vi "挥发酚测量数据储存.vi"   [LabVIEW 2016, in "挥发酚.lvlib"]
uses:
  <vilib>/ptbypt/NI_PtbyPt.lvlib
types:
  T1 = cluster{"时间标识":timestamp, "监测值":sgl, "单位":u16, "数据标识":string, "因子编码":u32, "标样参考值":sgl, "X0":sgl, "X^2":sgl, "X":sgl, "B 2":sgl, "跨度值":sgl, "量程":sgl}
  T2 = enum16{"维护数据", "水样测试", "标样核查", "零点核查", "跨度核查", "空白测试", "平行样测试", "加标回收", "空白校准", "标样校准", "初始化（清洗）"}
  T3 = cluster{"系统时间":timestamp, "工作状态":u16, "测量模式":enum16{"待机", "连续模式", "周期模式", "定点模式", "受控模式", "手动模式"}, "告警代码":u16, "故障代码":u16, "日志代码":u16, "软件版本":u16, "测量间隔":u16, "消解实时温度":dbl, "校准间隔（天）":u16, "校准间隔（时）":u16, "周期测量时间（23_16）":u16, "周期测量时间（15_0）":u16, "清洗周期（次数）":u16, "运行模式":u16, "自动校准状态":u16, "自动清洗状态":u16}
  T4 = enum16{"水样测试", "标样核查", "跨度核查", "零点核查", "空白测试", "平行样测试", "加标回收", "空白校准", "标样1校准", "标样2校准"}[]
  T5 = cluster{"运行模式":enum16{"维护模式", "常规模式", "应急模式", "质控模式", "性能测试"}, "质控频次":enum16{"关闭", "每天", "星期一", "星期二", "星期三", "星期四", "星期五", "星期六", "星期日"}, "空白核查时间":u16, "跨度核查时间":u16, "测量间隔":u16}
  T6 = cluster{"因子编码":u32, "单位":u16, "标样2参考值":sgl, "水样数据时间":timestamp, "水样实测值":sgl, "水样数据标识":string, "标样2数据时间":timestamp, "标样2实测值":sgl, "标样2数据标识":string, "空白数据时间":timestamp, "空白实测值":sgl, "空白数据标识":string, "零点核查数据时间":timestamp, "零点核查实测值":sgl, "零点核查数据标识":string, "跨度核查数据时间":timestamp, "跨度核查实测值":sgl, "跨度核查数据标识":string, "加标回收数据时间":timestamp, "加标回收实测值":sgl, "加标回收数据标识":string, "平行样数据时间":timestamp, "平行样实测值":sgl, "平行样数据标识":string, "标样1参考值":sgl, "标样1数据时间":timestamp, "标样1实测值":sgl, "标样1数据标识":string, "标样核查数据时间":timestamp, "标样核查实测值":sgl, "标样核查数据标识":string}
  T7 = cluster{"跨度值":dbl, "零点标准液浓度":dbl, "跨度标准液浓度":dbl, "标准液标准浓度":dbl, "零点标准液偏差":dbl, "跨度标准液偏差":dbl, "标准液标准偏差":dbl}
  T8 = cluster{"水样数据时间":timestamp, "空白数据时间":timestamp, "零点核查数据时间":timestamp, "跨度核查数据时间":timestamp, "加标回收数据时间":timestamp, "平行样数据时间":timestamp, "标样核查数据时间":timestamp, "标样1数据时间":timestamp, "标样2数据时间":timestamp}
  T9 = cluster{"公式":cluster{"X^2":dbl, "X":dbl, "B":dbl}, "校准":cluster{"校准？":bool, "校准点1-5":u16, "校准浓度":dbl}}
  T10 = cluster{"测量精度":u16, "消解温度":u16, "消解时长":u16, "量程下限":sgl, "量程上限":sgl, "曲线斜率K":sgl, "曲线斜率B":sgl, "标定日期":timestamp, "标液1浓度":sgl, "标液1测量过程值":sgl, "标液2浓度":sgl, "标液2测量过程值":sgl, "标液3浓度":sgl, "标液3测量过程值":sgl, "标液4浓度":sgl, "标液4测量过程值":sgl, "标液5浓度":sgl, "标液5测量过程值":sgl, "线性相关系数":sgl, "试剂余量":u32, "测量滴定值或吸光度":sgl, "标样2校准时间":timestamp, "检出限值":sgl, "校准系数":sgl, "设备系列号":string, "显色温度":u16, "显色时间":u16, "试剂余量1":u16, "试剂余量2":u16, "试剂余量3":u16, "试剂余量4":u16, "试剂余量5":u16, "试剂余量6":u16, "试剂余量7":u16, "试剂余量8":u16, "试剂余量9":u16, "试剂余量10":u16, "当前量程低位":sgl, "当前量程高位":sgl}
  T11 = cluster{"测量量程":sgl, "测量检出限":sgl, "测量精度":sgl, "测量间隔":sgl, "消解温度":sgl, "消解时长":sgl, "三项式系数":sgl, "二次多项式系数":sgl, "曲线斜率":sgl, "曲线截距":sgl, "线性相关系数":sgl, "空白校准时间":timestamp, "标样校准时间":timestamp, "测量信号值":sgl, "稀释倍数":sgl, "量程系数":sgl}
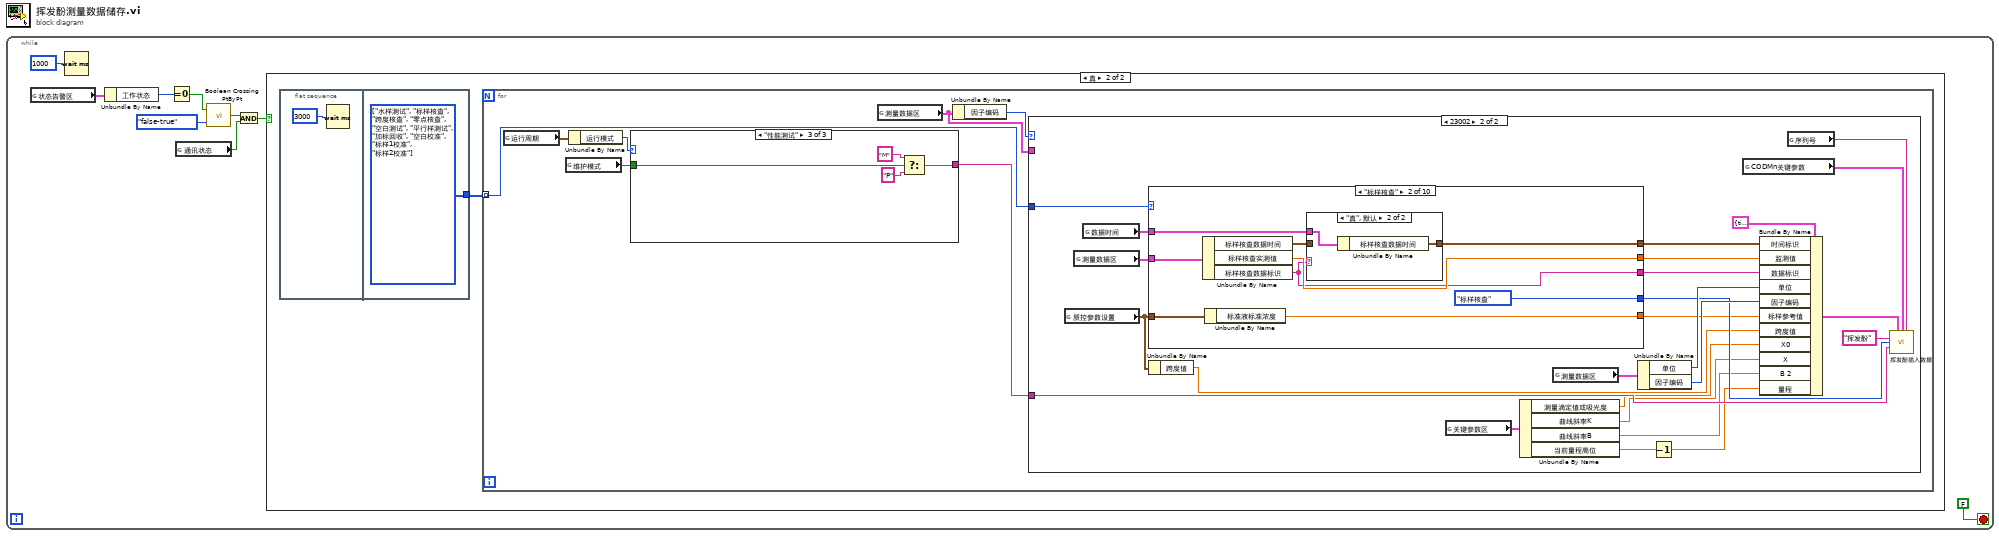
[diagram p0: block diagram]
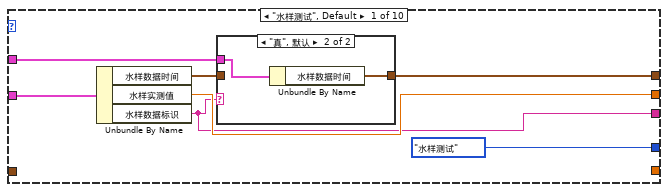
[diagram p4: hidden frame]
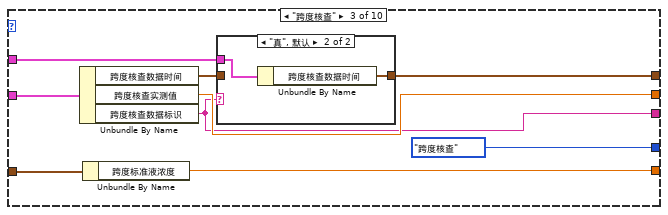
[diagram p7: hidden frame]
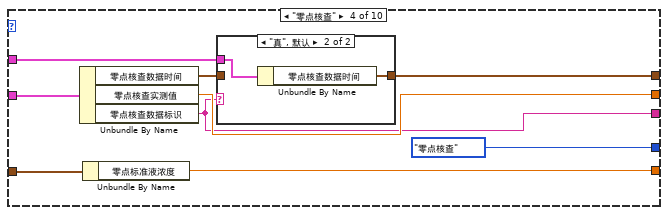
[diagram p9: hidden frame]
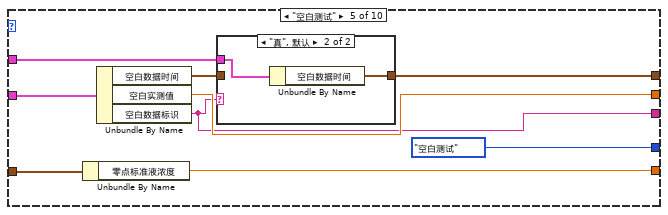
[diagram p11: hidden frame]
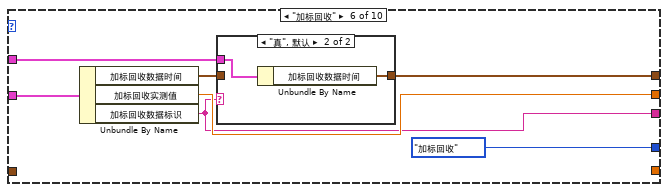
[diagram p13: hidden frame]
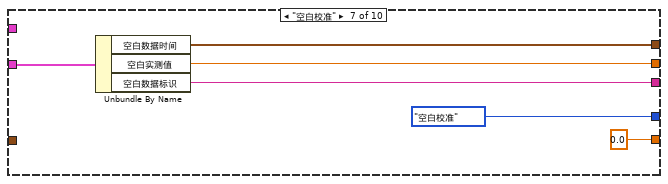
[diagram p15: hidden frame]
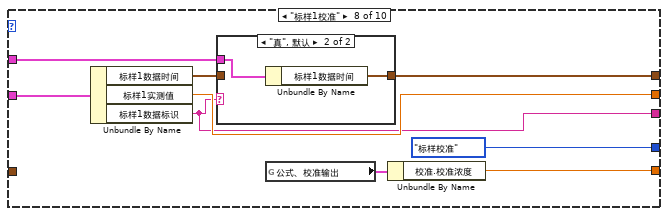
[diagram p16: hidden frame]
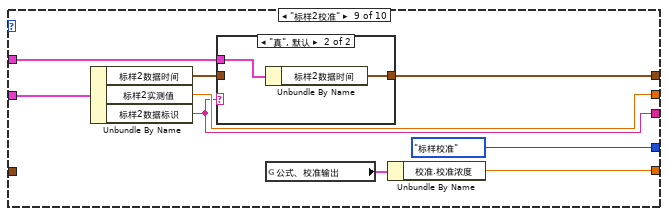
[diagram p18: hidden frame]
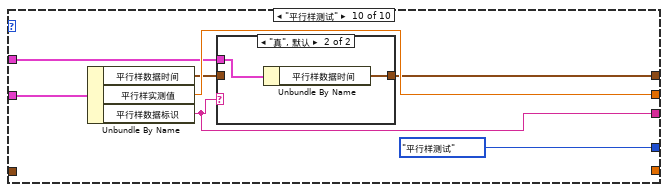
[diagram p20: hidden frame]
diagram:
  n1 = while {
    stop <- FALSE stop-if-true
    n2 = global read "VAR挥发酚全局变量.vi" "状态告警区"() -> (w5:T3)
    n3 = Wait (ms)(milliseconds to wait=u32 1000 ("等待时间（毫秒）")) -> ()  [unwired: 1 out]
    n4 = Unbundle By Name(w5) -> ("工作状态"=w4:u16)
    n5 = Equal To 0?(x=w4) -> (x = 0?=w6:bool)
    n6 = global read "VAR挥发酚全局变量.vi" "通讯状态"() -> (w2:bool)
    n7 = call <vilib>:"Boolean Crossing PtByPt.vi"("direction"=enum16{"either", "false-true", "true-false"}."false-true", "input"=w6) -> ("crossing"=w3:bool)  [unwired: 1 in]
    n8 = And(x=w3, y=w2) -> (x .and. y?=w1:bool)
    n9 = case shown="真" w1 {
      frame False {
      }
      frame True {
        n10 = flat-sequence {
          tunnel: [w12] -> w10
          frame #0 {
            n11 = Wait (ms)(milliseconds to wait=u32 3000 ("等待时间（毫秒）")) -> ()  [unwired: 1 out]
          }
          frame #1 {
            w12 = T4 [enum."水样测试", enum."标样核查", enum."跨度核查", enum."零点核查", enum."空白测试", enum."平行样测试", enum."加标回收", enum."空白校准", enum."标样1校准", enum."标样2校准"] items=["水样测试", "标样核查", "跨度核查", "零点核查", "空白测试", "平行样测试", "加标回收", "空白校准", "标样1校准", "标样2校准"]
          }
        }
        n12 = for {
          tunnel: w10 -> [w18] mode=indexing
          n13 = global read "挥发酚断电保存全局变量.vi" "运行周期"() -> (w17:T5)
          n14 = global read "挥发酚断电保存全局变量.vi" "维护模式"() -> (w13:bool)
          n15 = Unbundle By Name(w17) -> ("运行模式"=w14:enum16{"维护模式", "常规模式", "应急模式", "质控模式", "性能测试"})
          n16 = case shown="\"性能测试\"" w14 {
            tunnel: ["M" ("数据标记表") w154 w162] -> w19
            tunnel: w13 -> [_ w157 w164]
            frame "维护模式" {
            }
            frame "常规模式", Default {
              n17 = global read "VAR挥发酚全局变量.vi" "手动启动"() -> (w158:bool)
              n18 = case shown="假" w158 {
                tunnel: ["N" ("数据标记表") "hd" ("数据标记表")] -> w156
                frame False {
                }
                frame True {
                }
              }
              n19 = Select(t="M", s=w157, f=w156) -> (s? t:f=w154:string)
            }
            frame "性能测试" {
              n20 = Select(t="M", s=w164, f="P") -> (s? t:f=w162:string)
            }
          }
          n21 = global read "VAR挥发酚全局变量.vi" "测量数据区"() -> (w16:T6)
          n22 = Unbundle By Name(w16) -> ("因子编码"=w15:u32)
          n23 = case shown="23002" w15 {
            tunnel: w16 -> [_ _]
            tunnel: w19 -> [_ w34]
            tunnel: w18 -> [_ w33]
            frame Default {
            }
            frame 23002 {
              n24 = global read "挥发酚断电保存全局变量.vi" "质控参数设置"() -> (w30:T7)
              n25 = global read "VAR挥发酚全局变量.vi" "测量数据区"() -> (w44:T6)
              n26 = global read "挥发酚断电保存全局变量.vi" "数据时间"() -> (w22:T8)
              n27 = case shown="\"标样核查\"" w33 {
                tunnel: w44 -> [w51 w63 w75 w87 w99 w109 w118 w127 w139 w148]
                tunnel: [w45 w55 w69 w81 w91 w103 w117 w121 w131 w143] -> w37
                tunnel: [w49 w62 w74 w86 w98 w107 w116 w126 w138 w147] -> w38
                tunnel: [w47 w57 w67 w79 w93 w106 w115 w119 w134 w145] -> w39
                tunnel: [T2."水样测试" ("测量模式") T2."标样核查" ("测量模式") T2."跨度核查" ("测量模式") T2."零点核查" ("测量模式") T2."空白测试" ("测量模式") T2."加标回收" ("测量模式") T2."空白校准" ("测量模式") T2."标样校准" ("测量模式") T2."标样校准" ("测量模式") T2."平行样测试" ("测量模式")] -> w36
                tunnel: w30 -> [_ w59 w72 w84 w95 _ _ _ _ _]
                tunnel: [_ w60 w71 w83 w96 _ 0.0 ("零点标准液浓度") w124 w136 _] -> w32
                tunnel: w22 -> [w48 w58 w68 w80 w94 w105 _ w122 w132 w146]
                frame "水样测试", Default {
                  n28 = Unbundle By Name(w51) -> ("水样数据时间"=w46:timestamp, "水样实测值"=w49:sgl, "水样数据标识"=w47:string)
                  n29 = case shown="\"真\", 默认" w47 {
                    tunnel: w48 -> [_ w54]
                    tunnel: w46 -> [w52 _]
                    tunnel: [w52 w53] -> w45
                    frame "N" {
                    }
                    frame "真", Default {
                      n30 = Unbundle By Name(w54) -> ("水样数据时间"=w53:timestamp)
                    }
                  }
                }
                frame "标样核查" {
                  n31 = Unbundle By Name(w63) -> ("标样核查数据时间"=w56:timestamp, "标样核查实测值"=w62:sgl, "标样核查数据标识"=w57:string)
                  n32 = Unbundle By Name(w59) -> ("标准液标准浓度"=w60:dbl)
                  n33 = case shown="\"真\", 默认" w57 {
                    tunnel: w58 -> [_ w66]
                    tunnel: w56 -> [w64 _]
                    tunnel: [w64 w65] -> w55
                    frame "N" {
                    }
                    frame "真", Default {
                      n34 = Unbundle By Name(w66) -> ("标样核查数据时间"=w65:timestamp)
                    }
                  }
                }
                frame "跨度核查" {
                  n35 = Unbundle By Name(w75) -> ("跨度核查数据时间"=w70:timestamp, "跨度核查实测值"=w74:sgl, "跨度核查数据标识"=w67:string)
                  n36 = Unbundle By Name(w72) -> ("跨度标准液浓度"=w71:dbl)
                  n37 = case shown="\"真\", 默认" w67 {
                    tunnel: w68 -> [_ w78]
                    tunnel: w70 -> [w76 _]
                    tunnel: [w76 w77] -> w69
                    frame "N" {
                    }
                    frame "真", Default {
                      n38 = Unbundle By Name(w78) -> ("跨度核查数据时间"=w77:timestamp)
                    }
                  }
                }
                frame "零点核查" {
                  n39 = Unbundle By Name(w87) -> ("零点核查数据时间"=w82:timestamp, "零点核查实测值"=w86:sgl, "零点核查数据标识"=w79:string)
                  n40 = Unbundle By Name(w84) -> ("零点标准液浓度"=w83:dbl)
                  n41 = case shown="\"真\", 默认" w79 {
                    tunnel: w80 -> [_ w90]
                    tunnel: w82 -> [w88 _]
                    tunnel: [w88 w89] -> w81
                    frame "N" {
                    }
                    frame "真", Default {
                      n42 = Unbundle By Name(w90) -> ("零点核查数据时间"=w89:timestamp)
                    }
                  }
                }
                frame "空白测试" {
                  n43 = Unbundle By Name(w95) -> ("零点标准液浓度"=w96:dbl)
                  n44 = Unbundle By Name(w99) -> ("空白数据时间"=w92:timestamp, "空白实测值"=w98:sgl, "空白数据标识"=w93:string)
                  n45 = case shown="\"真\", 默认" w93 {
                    tunnel: w94 -> [_ w102]
                    tunnel: w92 -> [w100 _]
                    tunnel: [w100 w101] -> w91
                    frame "N" {
                    }
                    frame "真", Default {
                      n46 = Unbundle By Name(w102) -> ("空白数据时间"=w101:timestamp)
                    }
                  }
                }
                frame "加标回收" {
                  n47 = Unbundle By Name(w109) -> ("加标回收数据时间"=w104:timestamp, "加标回收实测值"=w107:sgl, "加标回收数据标识"=w106:string)
                  n48 = case shown="\"真\", 默认" w106 {
                    tunnel: w105 -> [_ w112]
                    tunnel: w104 -> [w110 _]
                    tunnel: [w110 w111] -> w103
                    frame "N" {
                    }
                    frame "真", Default {
                      n49 = Unbundle By Name(w112) -> ("加标回收数据时间"=w111:timestamp)
                    }
                  }
                }
                frame "空白校准" {
                  n50 = Unbundle By Name(w118) -> ("空白数据时间"=w117:timestamp, "空白实测值"=w116:sgl, "空白数据标识"=w115:string)
                }
                frame "标样1校准" {
                  n51 = Unbundle By Name(w127) -> ("标样1数据时间"=w120:timestamp, "标样1实测值"=w126:sgl, "标样1数据标识"=w119:string)
                  n52 = case shown="\"真\", 默认" w119 {
                    tunnel: w122 -> [_ w130]
                    tunnel: w120 -> [w128 _]
                    tunnel: [w128 w129] -> w121
                    frame "N" {
                    }
                    frame "真", Default {
                      n53 = Unbundle By Name(w130) -> ("标样1数据时间"=w129:timestamp)
                    }
                  }
                  n54 = global read "挥发酚断电保存全局变量.vi" "公式、校准输出"() -> (w123:T9)
                  n55 = Unbundle By Name(w123) -> ("校准.校准浓度"=w124:dbl)
                }
                frame "标样2校准" {
                  n56 = Unbundle By Name(w139) -> ("标样2数据时间"=w133:timestamp, "标样2实测值"=w138:sgl, "标样2数据标识"=w134:string)
                  n57 = case shown="\"真\", 默认" w134 {
                    tunnel: w132 -> [_ w142]
                    tunnel: w133 -> [w140 _]
                    tunnel: [w140 w141] -> w131
                    frame "N" {
                    }
                    frame "真", Default {
                      n58 = Unbundle By Name(w142) -> ("标样2数据时间"=w141:timestamp)
                    }
                  }
                  n59 = global read "挥发酚断电保存全局变量.vi" "公式、校准输出"() -> (w135:T9)
                  n60 = Unbundle By Name(w135) -> ("校准.校准浓度"=w136:dbl)
                }
                frame "平行样测试" {
                  n61 = Unbundle By Name(w148) -> ("平行样数据时间"=w144:timestamp, "平行样实测值"=w147:sgl, "平行样数据标识"=w145:string)
                  n62 = case shown="\"真\", 默认" w145 {
                    tunnel: w146 -> [_ w152]
                    tunnel: w144 -> [w150 _]
                    tunnel: [w150 w151] -> w143
                    frame "N" {
                    }
                    frame "真", Default {
                      n63 = Unbundle By Name(w152) -> ("平行样数据时间"=w151:timestamp)
                    }
                  }
                }
              }
              n64 = Unbundle By Name(w30) -> ("跨度值"=w29:dbl)
              n65 = global read "VAR挥发酚全局变量.vi" "关键参数区"() -> (w26:T10)
              n66 = Unbundle By Name(w26) -> ("测量滴定值或吸光度"=w25:sgl, "曲线斜率K"=w24:sgl, "曲线斜率B"=w23:sgl, "当前量程高位"=w21:sgl)
              n67 = global read "VAR挥发酚全局变量.vi" "测量数据区"() -> (w41:T6)
              n68 = Unbundle By Name(w41) -> ("单位"=w43:u16, "因子编码"=w42:u32)
              n69 = Decrement(x=w21) -> (x-1=w20:sgl)
              n70 = global read "挥发酚断电保存全局变量.vi" "CODMn关键参数"() -> (w31:T11)
              n71 = Bundle By Name(cluster=T1 {"时间标识"=timestamp(0 s since 1904-01-01), "监测值"=0.0, "单位"=0, "数据标识"="", "因子编码"=0, "标样参考值"=0.0, "X0"=0.0, "X^2"=0.0, "X"=0.0, "B 2"=0.0, "跨度值"=0.0, "量程"=0.0} ("data"), "时间标识"=w37, "监测值"=w38, "数据标识"=w39, "单位"=w43, "因子编码"=w42, "标样参考值"=w32, "跨度值"=w29, "X0"=w25, "X"=w24, "B 2"=w23, "量程"=w20) -> (w27:T1)
              n72 = global read "VAR挥发酚全局变量.vi" "序列号"() -> (w40:string)
              n73 = call "挥发酚插入数据.vi"("data"=w27, "挥发酚关键参数"=w31, "SN"=w40, "table"="挥发酚", "测量模式"=w36, "数据类型"=w34) -> ()  [unwired: 9 in, 1 out]
            }
          }
        }
      }
    }
  }
